vi "logrecordstringarray2D.vi"(7 "logsetting":enum16{"error", "info", "debug"}(ring), 8 "error in":errorcluster, 9 "logtype":enum16{"error", "info", "debug"}(ring), 10 "LogPath":path, 11 "Msg":string[][](array[string])) -> (0 "error out":errorcluster)   [LabVIEW 2011]
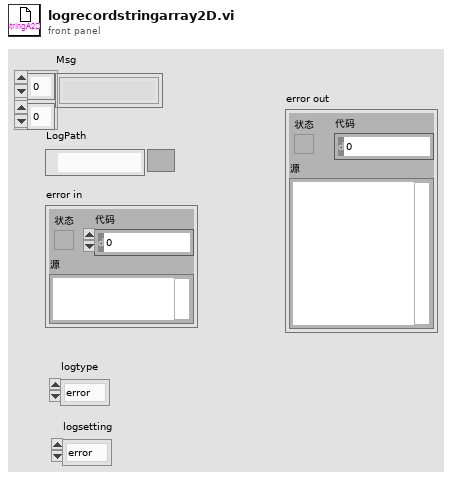
[diagram p1: front panel]
types:
  T1 = enum16{"open", "replace", "create", "open or create", "replace or create", "replace or create with confirmation"}
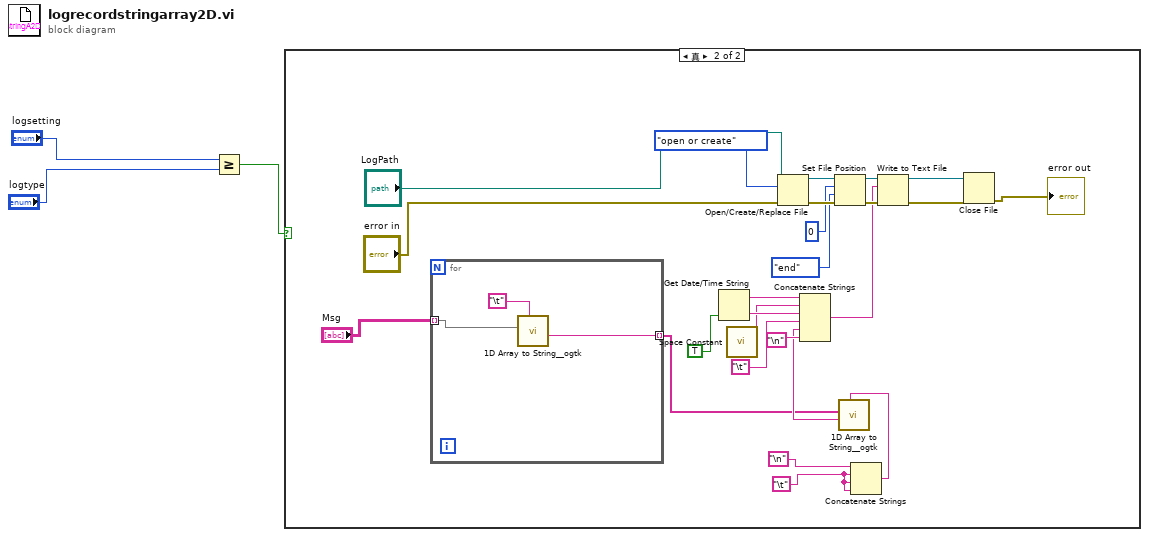
[diagram p0: block diagram]
diagram:
  n1 = Greater Or Equal?(x="logsetting", y="logtype") -> (x >= y?=w1:bool)
  n2 = case shown="真" w1 {
    frame False {
    }
    frame True {
      w7 = "\t"
      n3 = for {
        tunnel: "Msg" -> [w31] mode=indexing
        tunnel: [w29] -> w4 mode=indexing
        n4 = call <userlib>:"1D Array to String__ogtk.vi"("delimiter (Tab)"="\t", "Array of Strings"=w31) -> ("delimited string"=w29:string)  [unwired: 9 in]
      }
      n5 = Get Date/Time String(want seconds? (F)=TRUE ("需要秒？(F)")) -> (date string=w15:string, time string=w17:string)  [unwired: 2 in]
      n6 = call <vilib>:"Space Constant.vi"() -> ("String"=w16:string)
      n7 = Open/Create/Replace File(file path (use dialog)="LogPath", error in="error in", operation (0:open)=T1."open or create" ("操作(0:open)")) -> (refnum out=w11:refnum<file>, error out=w21:errorcluster)  [unwired: 3 in, 1 out]
      n8 = Set File Position(offset (in bytes) (0)=i64 0 ("偏移量（字节）（0）"), refnum=w11, from (0:start)=enum16{"start", "end", "current"}."end" ("自（0:起始）"), error in=w21) -> (refnum out=w13:refnum<file>, error out=w22:errorcluster)
      n9 = Concatenate Strings("\n", w7, w7, w7) -> (w8:string)
      n10 = call <userlib>:"1D Array to String__ogtk.vi"("delimiter (Tab)"=w8, "Array of Strings"=w4) -> ("delimited string"=w10:string)  [unwired: 9 in]
      n11 = Concatenate Strings(w15, w16, w17, "\t", w10, "\n") -> (w19:string)
      n12 = Write to Text File(file (use dialog)=w13, text=w19, error in=w22) -> (refnum out=w24:refnum<file>, error out=w25:errorcluster)  [unwired: 1 in, 1 out]
      n13 = Close File(refnum=w24, error in=w25) -> (error out=→"error out":errorcluster)  [unwired: 1 out]
    }
  }
